vi "subPrintDebugInfo.vi"(11 "Dependency List":T1) -> (3 "spreadsheet string":string)   [LabVIEW 2020, in "DependencyInspection.lvlib" / "CDependencyInspection.lvclass"]
uses:
  CDependencyInspection.lvclass
  CDependencyList/DependencyList.ctl
  obj/Addons/LabVIEWObjectInterfaces.lvlibp/LabVIEWObjectInterfaces/ILabVIEWItem/ILabVIEWItem.lvclass
  CDependencyList/CDependencyList.lvclass
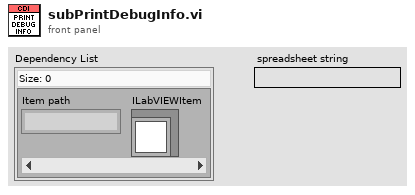
[diagram p1: front panel]
types:
  T1 = typedef "DependencyInspection.lvlib/CDependencyList.lvclass/DependencyList.ctl" = map{string, refnum<class "ILabVIEWItem.lvclass">}
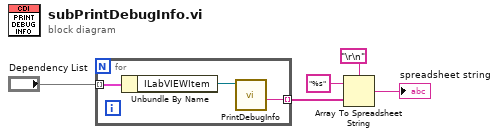
[diagram p0: block diagram]
diagram:
  n1 = for {
    tunnel: "Dependency List" -> [w8] mode=indexing
    tunnel: [w6] -> w2 mode=indexing
    n2 = Unbundle By Name(w8) -> ("ILabVIEWItem"=w7:refnum<class "ILabVIEWItem.lvclass">)
    n3 = call-dynamic "PrintDebugInfo.vi"("ILabVIEWItem in"=w7) -> ("Debug string"=w6:string)  [unwired: 8 in, 2 out]
  }
  n4 = Array To Spreadsheet String(delimiter (Tab)="\r\n", array=w2, 3:"%s" ("format string")) -> (spreadsheet string=→"spreadsheet string":string)
